vi "Set_5G_Carrier_Bandwidth.vi"(8 "error in (no error)":errorcluster, 10 "value":string(combo)="0", 11 "Base Station":T1) -> (0 "error out":errorcluster, 3 "Output String":string)   [LabVIEW 2021]
uses:
  Controls/Base_Station_Emulator.ctl
  Controls/TCP_FGV.ctl
panel:
  # "the possible values are 10,20,25,30,40,50 \n If subcarrier_spacing is 1, then the possible values are \n10,20,30,40,50,60,80,100. \n The default value is 0."
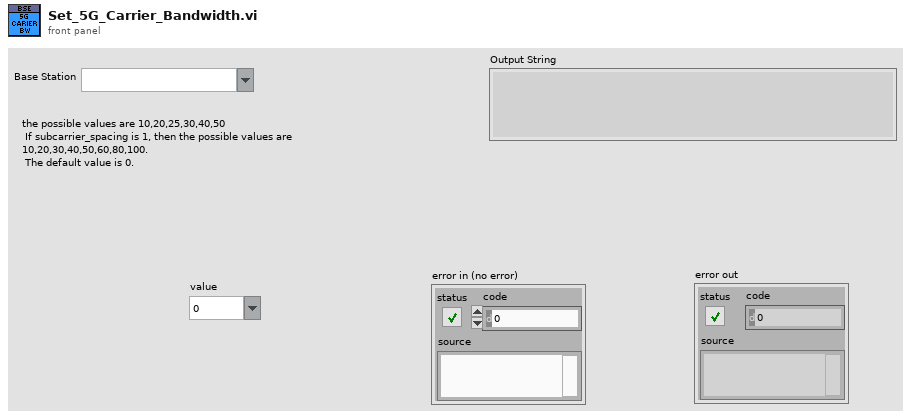
[diagram p1: front panel]
types:
  T1 = typedef "Base_Station_Emulator.ctl" = string
  T2 = typedef "TCP_FGV.ctl" = enum16{"Open", "Read", "Write", "Close"}
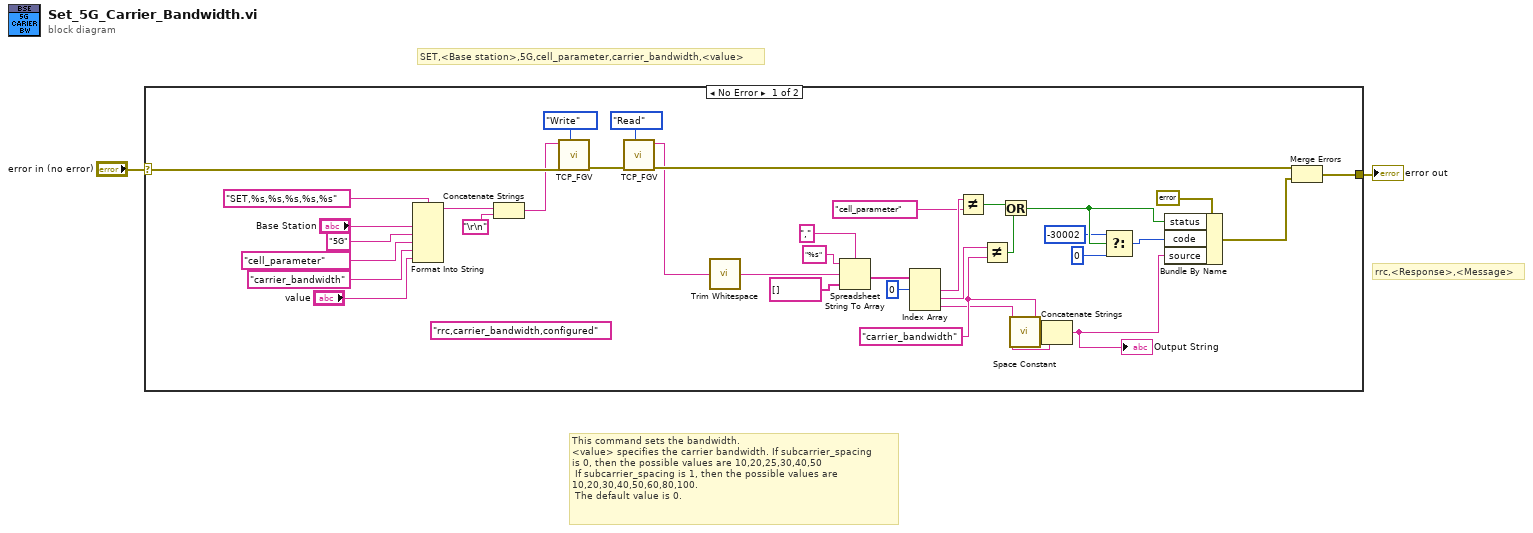
[diagram p0: block diagram]
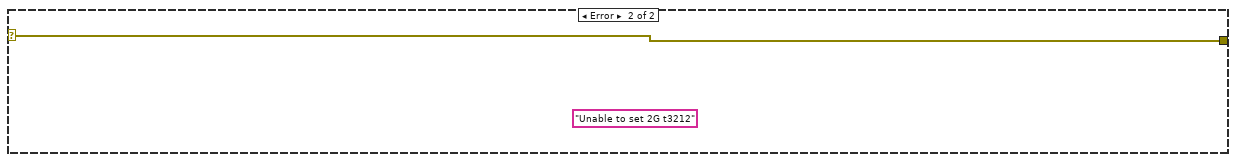
[diagram p2: hidden frame]
diagram:
  # "This command sets the bandwidth. \n<value> specifies the carrier bandwidth. If subcarrier_spacing \nis 0, then the possible values are 10,20,25,30,40,50 \n If subcarrier_spacing is 1, then the possible values are \n10,20,30,40,50,60,80,100. \n The default value is 0."
  # "SET,<Base station>,5G,cell_parameter,carrier_bandwidth,<value>"
  # "rrc,<Response>,<Message>"
  n1 = case shown="No Error" "error in (no error)" {
    selector: "error in (no error)" -> [w36 w40]
    tunnel: [w14 w40] -> w1
    frame No Error {
      (unwired) "rrc,carrier_bandwidth,configured" ("format string")
      w12 = "carrier_bandwidth"
      n2 = Format Into String(format string="SET,%s,%s,%s,%s,%s", "Base Station", "5G", "cell_parameter", "carrier_bandwidth", "value") -> (resulting string=w6:string)  [unwired: 2 in, 1 out]
      n3 = Concatenate Strings(w6, "\r\n") -> (w5:string)
      n4 = call "TCP_FGV.vi"("Command"=w5, "error in (no error)"=w36, "Operation"=TCP_FGV."Write") -> ("error out"=w15:errorcluster)  [unwired: 6 in, 1 out]
      n5 = call "TCP_FGV.vi"("error in (no error)"=w15, "Operation"=TCP_FGV."Read") -> ("Data Out"=w4:string, "error out"=w17:errorcluster)  [unwired: 7 in]
      n6 = call <vilib>:"Trim Whitespace.vi"("string"=w4) -> ("trimmed string"=w31:string)  [unwired: 1 in]
      n7 = Spreadsheet String To Array(delimiter (Tab)=",", format string="%s", spreadsheet string=w31, array type (2D Dbl)=string[] []) -> (array=w27:string[])
      n8 = Index Array(array=w27, index #1=0 ("index")) -> (element #1=w28:string, element #2=w18:string, element #3=w11:string)  [unwired: 2 in]
      n9 = Not Equal?(x=w28, y="cell_parameter" ("format string")) -> (x != y?=w29:bool)
      n10 = Not Equal?(x=w18, y=w12) -> (x != y?=w30:bool)
      n11 = Or(x=w29, y=w30) -> (x .or. y?=w32:bool)
      n12 = call <vilib>:"Space Constant.vi"() -> ("String"=w13:string)
      n13 = Concatenate Strings(w12, w13, w11) -> (w10:string)
      "Output String" <- w10
      n14 = Select(t=-30002 ("code"), s=w32, f=0 ("code")) -> (s? t:f=w33:i32)
      n15 = Bundle By Name(cluster=errorcluster {"status"=FALSE, "code"=0, "source"=""} ("error constant"), "status"=w32, "code"=w33, "source"=w10) -> (w16:errorcluster)
      n16 = Merge Errors(w17, w16) -> (w14:errorcluster)
    }
    frame Error {
      (unwired) "Unable to set 2G t3212" ("source")
    }
  }
  "error out" <- w1
